vi "Destroy.vi"(8 "error in":errorcluster, 11 "EDS in":refnum<class "EDS.lvclass">) -> (0 "error out":errorcluster, 3 "EDS out":refnum<class "EDS.lvclass">)   [LabVIEW 2024, in "EDS.lvlib" / "EDS.lvclass"]
uses:
  EDS.lvclass
  EDS.lvclass/EDS.ctl
  Sorted Object Dictionary/Sorted Object Dictionary.lvclass
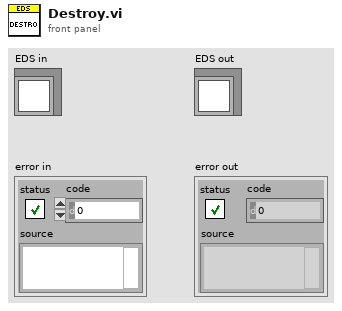
[diagram p1: front panel]
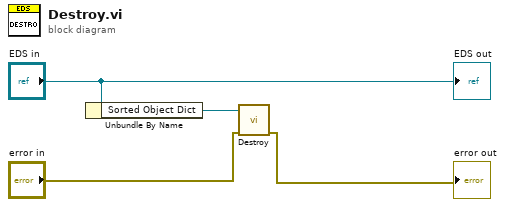
[diagram p0: block diagram]
diagram:
  n1 = Unbundle By Name("EDS in") -> ("Sorted Object Dict"=w3:refnum<class "Sorted Object Dictionary.lvclass">)
  n2 = call "Destroy.vi"("error in"="error in", "Sorted Object Dictionary in"=w3) -> ("error out"=→"error out":errorcluster)  [unwired: 8 in, 1 out]
  "EDS out" <- "EDS in"
